vi "ex_CreateError.vi"(8 "error in (no error)":errorcluster, 9 "source":string, 10 "code":i32, 11 "error?":bool) -> (0 "error out":errorcluster)   [LabVIEW 2017]
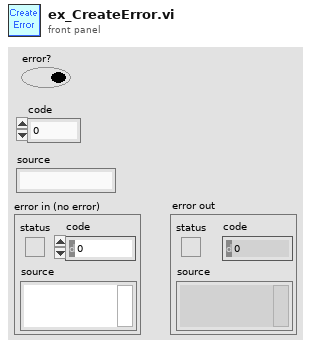
[diagram p1: front panel]
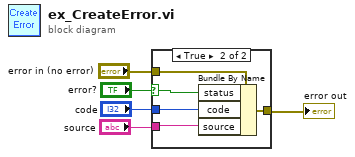
[diagram p0: block diagram]
diagram:
  n1 = case shown="True" "error?" {
    selector: "error?" -> [_ w7]
    tunnel: "error in (no error)" -> [w6 w11]
    tunnel: [w6 w10] -> w3
    tunnel: "code" -> [_ w9]
    tunnel: "source" -> [_ w8]
    frame False {
    }
    frame True {
      n2 = Bundle By Name(cluster=w11, "status"=w7, "code"=w9, "source"=w8) -> (w10:errorcluster)
    }
  }
  "error out" <- w3
